vi "SRE.vi"(8 "error in (no error)":errorcluster, 10 "Node In":string, 11 "VISA resource name":refnum<visa-resource-name>) -> (0 "error out":errorcluster, 1 "SRE":u8, 2 "Node Out":string, 3 "VISA resource name out":refnum<visa-resource-name>, 4 "Command String":string)   [LabVIEW 2012, in "Keithley 2600 Series.lvlib"]
doc: "Service Request Enable query. *SRE?\n\n<b>Functions and Attributes Used</b>\nstatus.request_enable"
uses:
  Keithley 2600 Series.lvlib
panel:
  # "(c) 2008 Keithley Instruments, Inc.  ALL RIGHTS RESERVED."
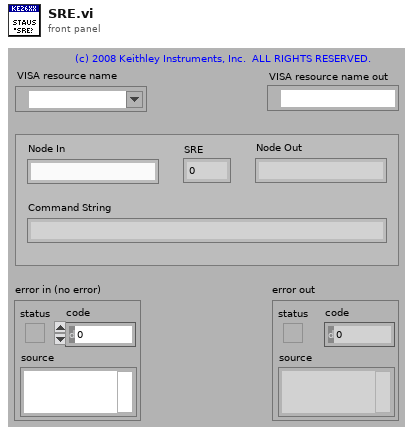
[diagram p1: front panel]
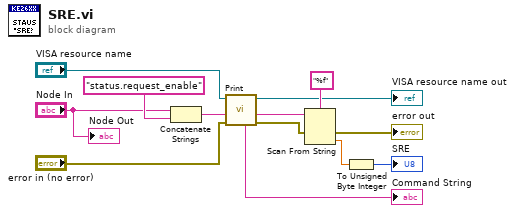
[diagram p0: block diagram]
diagram:
  n1 = Concatenate Strings("Node In", "status.request_enable" ("string")) -> (w8:string)
  n2 = call "Print.vi"("error in (no error)"="error in (no error)", "Input"=w8, "VISA resource name"="VISA resource name") -> ("error out"=w5:errorcluster, "Output"=w10:string, "VISA resource name out"=→"VISA resource name out":refnum<visa-resource-name>, "Command String"=→"Command String":string)  [unwired: 2 in, 3 out]
  n3 = Scan From String(format string="%f", input string=w10, error in=w5) -> (error out=→"error out":errorcluster, output 1=w3:dbl)  [unwired: 1 in, 3 out]
  n4 = To Unsigned Byte Integer(number=w3) -> (unsigned 8bit integer=→"SRE":u8)
  "Node Out" <- "Node In"
